vi "subGeneratePackets.vi"(0 "Samples per Symbol":i32, 1 "Packet Pad \n[samples]":i32, 3 "PSK system parameters":T2, 5 "Tx IQ Sampling\nRate [s/sec]":dbl, 7 "Pulse Shaping Filter Parameters":T3, 9 "Packet Repeat":i32, 11 "PN sequence order\nfor Sync Bits":i32, 12 "Packet Parameters":T1, 15 "Message Text":string) -> (4 "Number of Packets":i32, 6 "Packets":cluster{"t0":dbl, "dt":dbl, "Y":cdb[]}[](array[cluster]), 10 "Symbol Rate":dbl)   [LabVIEW 2015]
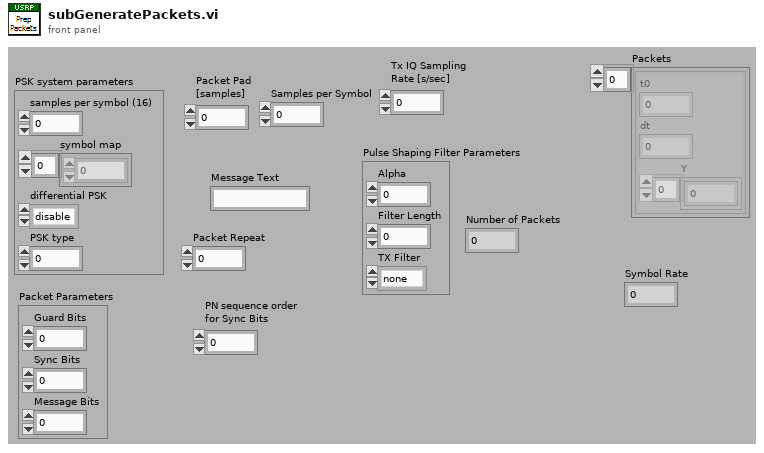
[diagram p1: front panel]
types:
  T1 = cluster{"Guard Bits ":i32, "Sync Bits":i32, "Message Bits":i32}
  T2 = cluster{"samples per symbol (16)":i32, "symbol map":cdb[], "differential PSK":enum16{"disable", "enable"}, "PSK type":u16}
  T3 = cluster{"Alpha":dbl, "Filter Length":i32, "TX Filter":enum16{"none", "Raised Cosine", "Root Raised Cos", "Gaussian"}}
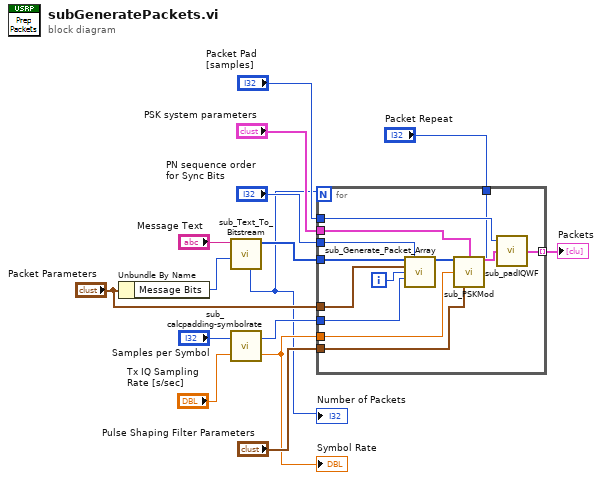
[diagram p0: block diagram]
diagram:
  n1 = Unbundle By Name("Packet Parameters") -> ("Message Bits"=w7:i32)
  n2 = call "sub_Text_To_Bitstream.vi"("Packet\nMessage Length (bits)"=w7, "text"="Message Text") -> ("message bitstream"=w11:i8[], "Number of Packets"=w2:i32)  [unwired: 7 in, 1 out]
  "Number of Packets" <- w2
  n3 = call "sub_calcpadding-symbolrate.vi"("Tx IQ Sampling\nRate [s/sec]"="Tx IQ Sampling\nRate [s/sec]", "Samples per Symbol"="Samples per Symbol") -> ("Symbol Rate"=w4:dbl, "Padding Bits"=w6:i32)
  "Symbol Rate" <- w4
  n4 = for {
    N: w2 -> [_]
    tunnel: "Packet Parameters" -> [w17]
    tunnel: [w22] -> w9 mode=indexing
    tunnel: w11 -> [w19]
    tunnel: "PN sequence order\nfor Sync Bits" -> [w27]
    tunnel: w6 -> [w18]
    tunnel: "PSK system parameters" -> [w25]
    tunnel: w4 -> [w24]
    tunnel: "Pulse Shaping Filter Parameters" -> [w23]
    tunnel: "Packet Pad \n[samples]" -> [w20]
    tunnel: "Packet Repeat" -> [w16]
    i -> [w28]
    n5 = call "sub_Generate_Packet_Array.vi"("user  bitstream"=w19, "PN sequence order\nfor Sync"=w27, "Packet Parameters"=w17, "Packet Number"=w28, "Cyclic Padding Bits"=w18) -> ("Output Packet"=w26:i8[])  [unwired: 10 in]
    n6 = call "sub_PSKMod.vi"("Packet to Transmit"=w26, "PSK system parameters"=w25, "Symbol Rate, Hz"=w24, "filter parameters"=w23) -> ("output complex waveform"=w21:cluster{"t0":dbl, "dt":dbl, "Y":cdb[]})  [unwired: 10 in, 1 out]
    n7 = call "sub_padIQWF.vi"("Repeat"=w16, "input complex waveform"=w21, "Packet Pad \n[samples]"=w20) -> ("output complex waveform"=w22:cluster{"t0":dbl, "dt":dbl, "Y":cdb[]})
  }
  "Packets" <- w9
